vi "Write Cursor Watch Plots.vi"(8 "error in (no error)":errorcluster, 10 "Watch Plots":i32[](array[numeric]), 11 "2D Plot.lvclass in":refnum<class "2D Plot.lvclass">) -> (0 "error out":errorcluster, 3 "2D Plot.lvclass out":refnum<class "2D Plot.lvclass">)   [LabVIEW 2017, in "2D Plot.lvclass"]
uses:
  <vilib>/Math Plots/2D Math Plots/2D Plot/2D Plot/2D Plot.lvclass
  <vilib>/Math Plots/2D Math Plots/2D Plot/2D Plot/2D Plot.lvclass/2D Plot.ctl
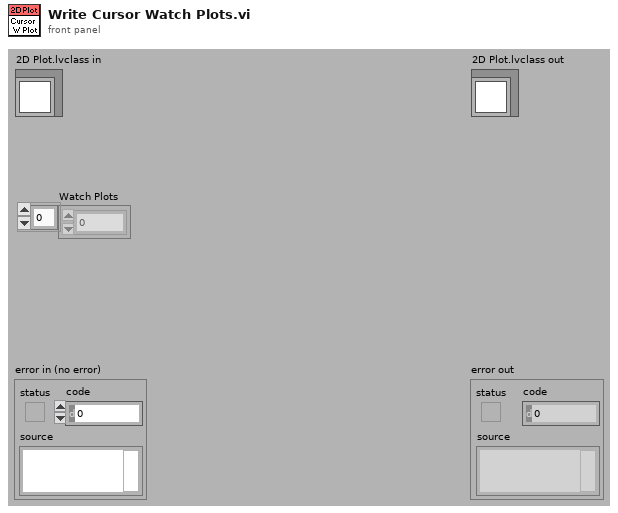
[diagram p1: front panel]
types:
  T1 = typedef "LVCursorListTypeDef.ctl" = cluster{"Name":string, "Color":u32, "Style":u8, "Point Style":u8, "Name Visible":bool, "Allow Drag":bool, "Cursor Mode":u32, "Plot":i32, "Index":i32, "Position":cluster{"X":dbl, "Y":dbl}, "X Scale":u32, "Y Scale":u32, "Watch Plots":i32[], "Watch All Plots":bool, "Plot Area":i32, "Label Offset":cluster{"X":dbl, "Y":dbl}}[]
  T2 = cluster{"Name":string, "Color":u32, "Style":u8, "Point Style":u8, "Name Visible":bool, "Allow Drag":bool, "Cursor Mode":u32, "Plot":i32, "Index":i32, "Position":cluster{"X":dbl, "Y":dbl}, "X Scale":u32, "Y Scale":u32, "Watch Plots":i32[], "Watch All Plots":bool, "Plot Area":i32, "Label Offset":cluster{"X":dbl, "Y":dbl}}
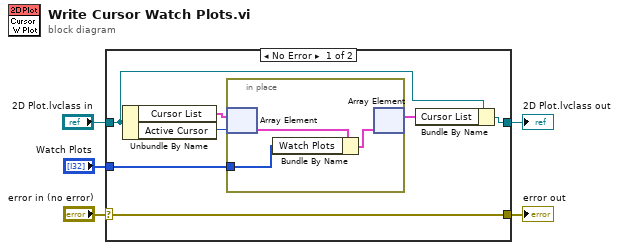
[diagram p0: block diagram]
diagram:
  n1 = case shown="No Error" "error in (no error)" {
    selector: "error in (no error)" -> [w12 w16]
    tunnel: "Watch Plots" -> [w8 _]
    tunnel: "2D Plot.lvclass in" -> [w7 w17]
    tunnel: [w6 w17] -> w4
    tunnel: [w12 w16] -> w2
    frame No Error {
      n2 = Unbundle By Name(w7) -> ("Cursor List"=w11:T1, "Active Cursor"=w9:i32)
      n3 = in-place {
        in-place-border: w8 -> [w14]
        n4 = in-place-array #1(w11, w9) -> (w15:T2)
        n5 = Bundle By Name(cluster=w15, "Watch Plots"=w14) -> (w13:T2)
        n6 = in-place-array #1(w13) -> (w10:T1)  [unwired: 1 out]
      }
      n7 = Bundle By Name(cluster=w7, "Cursor List"=w10) -> (w6:refnum<class "2D Plot.lvclass">)
    }
    frame Error {
    }
  }
  "error out" <- w2
  "2D Plot.lvclass out" <- w4
